vi "Sim_Yoke_Shin_TP059851_SPCC_Assignment_server.vi"() -> ()   [LabVIEW 2020]
uses:
  <vilib>/Utility/file.llb/Read Delimited Spreadsheet (string).vi
  <vilib>/Utility/file.llb/Write Delimited Spreadsheet (string).vi
panel:
  out "Amount out":string
  out "Data from Client":string
  out "error of functions":errorcluster
  out "error of login":errorcluster
  out "user input":string
  out "Output User Details":string
  out "User ID Array":string[](array[string])
  # "Server"
  # "Login"
  # "Functions"
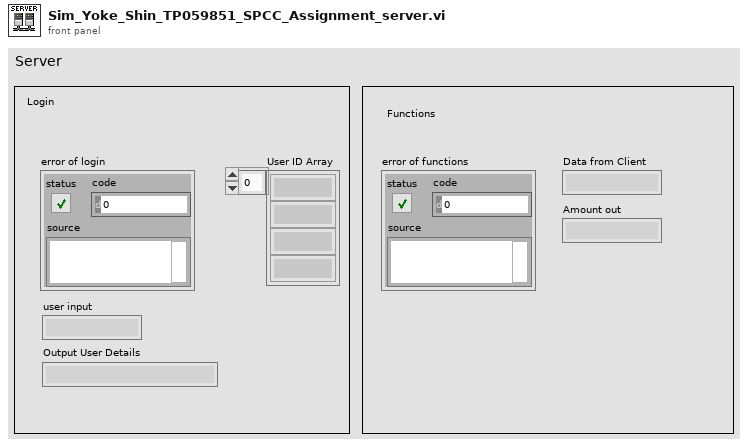
[diagram p1: front panel]
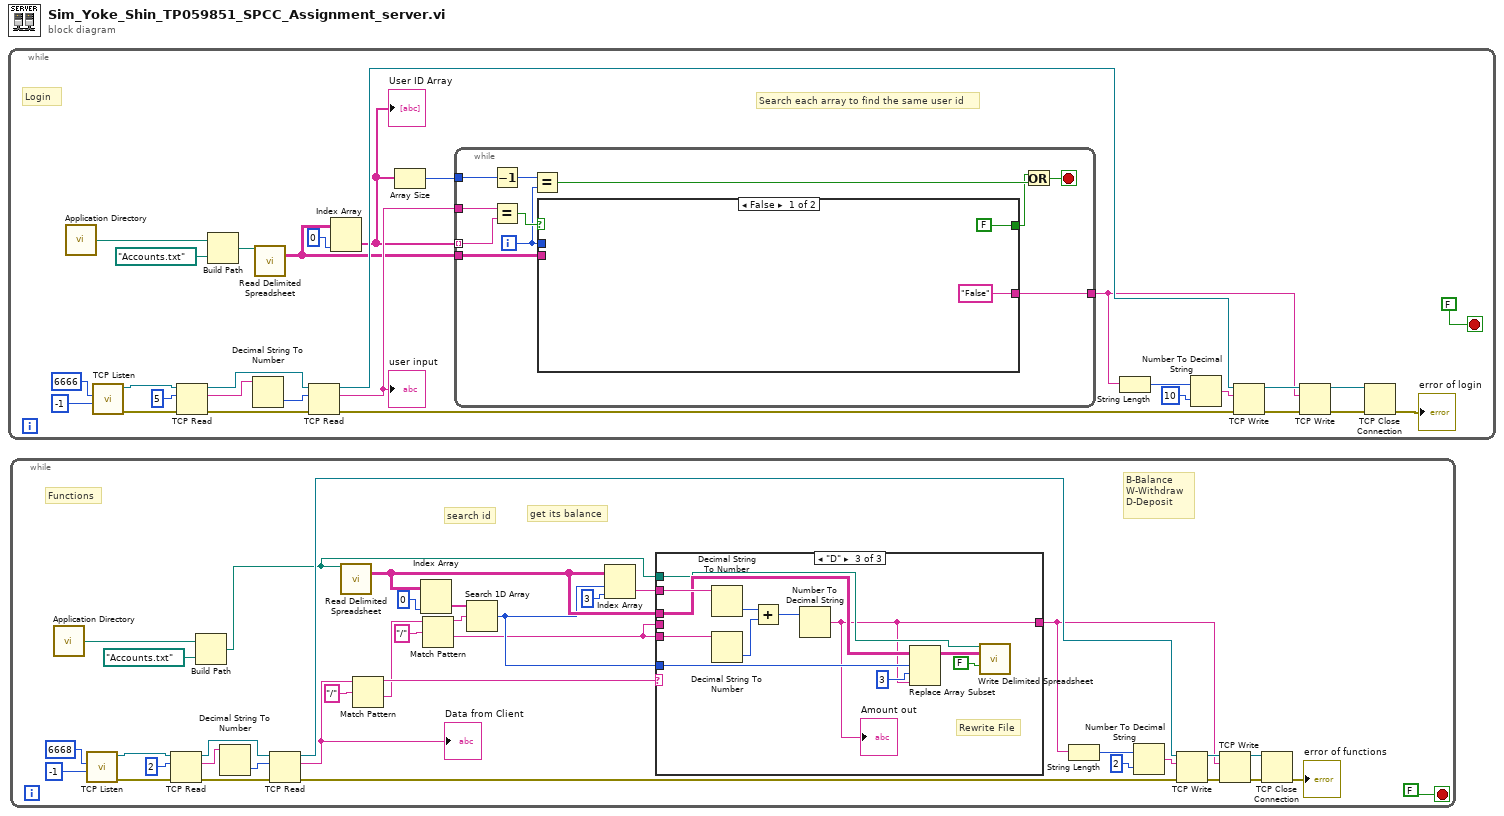
[diagram p0: block diagram]
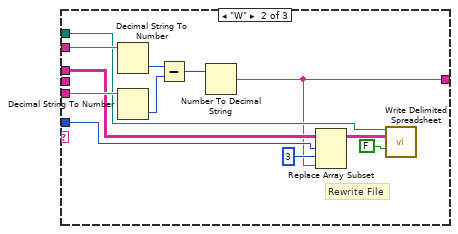
[diagram p3: hidden frame]
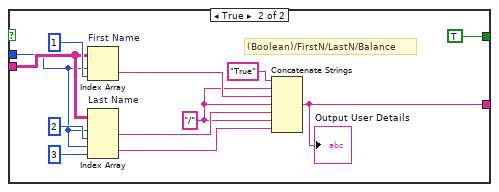
[diagram p4: hidden frame]
diagram:
  n1 = while {
    stop <- FALSE stop-if-true
    # "Search each array to find the same user id"
    # "Login"
    n2 = call <vilib>:"Application Directory.vi"() -> ("Application Directory"=w2:path)
    n3 = call <vilib>:"TCP Listen.vi"("timeout ms (wait forever: -1)"=-1, "port"=u16 6666) -> ("error out"=w20:errorcluster, "connection ID"=w29:refnum<k5>)  [unwired: 5 in, 3 out]
    n4 = TCP Read(connection ID=w29, bytes to read=5, error in (no error)=w20) -> (connection ID out=w28:refnum<k5>, data out=w18:string, error out=w21:errorcluster)  [unwired: 2 in]
    n5 = Build Path(base path=w2, name or relative path=path "Accounts.txt") -> (appended path=w1:path)
    n6 = Decimal String To Number(string=w18) -> (number=w17:i32)  [unwired: 2 in, 1 out]
    n7 = call-poly <vilib>:"Read Delimited Spreadsheet.vi"("file path (dialog if empty)"=w1) -> ("all rows"=w15:string[][])  [unwired: 9 in, 5 out]
    n8 = TCP Read(connection ID=w28, bytes to read=w17, error in (no error)=w21) -> (connection ID out=w27:refnum<k5>, data out=w16:string, error out=w22:errorcluster)  [unwired: 2 in]
    "user input" <- w16
    n9 = Index Array(array=w15, index (col)=0 ("disabled index (col)")) -> (element=w14:string[])  [unwired: 1 in]
    "User ID Array" <- w14
    n10 = Array Size(array=w14) -> (size(s)=w10:i32)
    n11 = while {
      tunnel: w14 -> [w33] mode=indexing
      tunnel: w16 -> [w39]
      tunnel: w15 -> [w38]
      tunnel: [w34] -> w13
      tunnel: w10 -> [w32]
      i -> [w36]
      stop <- w30 stop-if-true
      n12 = Decrement(x=w32) -> (x-1=w37:i32)
      n13 = Equal?(x=w39, y=w33) -> (x = y?=w40:bool)
      n14 = Equal?(x=w37, y=w36) -> (x = y?=w35:bool)
      n15 = case shown="False" w40 {
        tunnel: w38 -> [_ w47]
        tunnel: w36 -> [_ w46]
        tunnel: [FALSE TRUE] -> w31
        tunnel: ["False" w48] -> w34
        frame False {
        }
        frame True {
          w44 = "/" ("string")
          # "(Boolean)/FirstN/LastN/Balance"
          n16 = Index Array "First Name"(array=w47, index (row)=w46, index (col)=1 ("disabled index (col)")) -> (element=w50:string)
          n17 = Index Array "Last Name"(array=w47, index (row) #1=w46, index (col) #1=2 ("disabled index (col)"), index (row) #2=w46, index (col) #2=3 ("disabled index (col)")) -> (element #1=w49:string, element #2=w43:string)
          n18 = Concatenate Strings("True" ("string"), w44, w50, w44, w49, w44, w43) -> (w48:string)
          "Output User Details" <- w48
        }
      }
      n19 = Or(x=w31, y=w35) -> (x .or. y?=w30:bool)
    }
    n20 = String Length(string=w13) -> (length=w12:i32)
    n21 = Number To Decimal String(number=w12, width (-)=i16 10) -> (decimal integer string=w11:string)
    n22 = TCP Write(connection ID=w27, data in=w11, error in (no error)=w22) -> (connection ID out=w26:refnum<k5>, error out=w23:errorcluster)  [unwired: 1 in, 1 out]
    n23 = TCP Write(connection ID=w26, data in=w13, error in (no error)=w23) -> (connection ID out=w25:refnum<k5>, error out=w24:errorcluster)  [unwired: 1 in, 1 out]
    n24 = TCP Close Connection(connection ID=w25, error in (no error)=w24) -> (error out=→"error of login":errorcluster)  [unwired: 1 in, 1 out]
  }
  n25 = while {
    stop <- FALSE stop-if-true
    # "B-Balance\nW-Withdraw\nD-Deposit"
    # "Functions"
    # "get its balance"
    # "search id"
    n26 = call <vilib>:"Application Directory.vi"() -> ("Application Directory"=w58:path)
    n27 = call <vilib>:"TCP Listen.vi"("timeout ms (wait forever: -1)"=-1, "port"=u16 6668) -> ("error out"=w81:errorcluster, "connection ID"=w91:refnum<k5>)  [unwired: 5 in, 3 out]
    n28 = TCP Read(connection ID=w91, bytes to read=2, error in (no error)=w81) -> (connection ID out=w90:refnum<k5>, data out=w77:string, error out=w82:errorcluster)  [unwired: 2 in]
    n29 = Build Path(base path=w58, name or relative path=path "Accounts.txt") -> (appended path=w56:path)
    n30 = Decimal String To Number(string=w77) -> (number=w76:i32)  [unwired: 2 in, 1 out]
    n31 = TCP Read(connection ID=w90, bytes to read=w76, error in (no error)=w82) -> (connection ID out=w89:refnum<k5>, data out=w55:string, error out=w83:errorcluster)  [unwired: 2 in]
    "Data from Client" <- w55
    n32 = call-poly <vilib>:"Read Delimited Spreadsheet.vi"("file path (dialog if empty)"=w56) -> ("all rows"=w66:string[][])  [unwired: 9 in, 5 out]
    n33 = Match Pattern(string=w55, regular expression="/") -> (before substring=w73:string, after substring=w72:string)  [unwired: 1 in, 2 out]
    n34 = Index Array(array=w66, index (col)=0 ("disabled index (col)")) -> (element=w75:string[])  [unwired: 1 in]
    n35 = Match Pattern(string=w72, regular expression="/") -> (before substring=w70:string, after substring=w60:string)  [unwired: 1 in, 2 out]
    n36 = Search 1D Array(1D array=w75, element=w70) -> (index of element=w65:i32)  [unwired: 1 in]
    n37 = Index Array(array=w66, index (row)=w65, index (col)=3 ("disabled index (col)")) -> (element=w67:string)
    n38 = case shown="\"D\"" w73 {
      tunnel: w67 -> [w92 w99 w116]
      tunnel: w60 -> [_ _ _]
      tunnel: w66 -> [_ w97 w112]
      tunnel: w65 -> [_ w94 w111]
      tunnel: w56 -> [_ w95 w108]
      tunnel: [w92 w93 w106] -> w64
      tunnel: w60 -> [_ w98 w105]
      frame "B", Default {
      }
      frame "W" {
        # "Rewrite File"
        n39 = Decimal String To Number(string=w99) -> (number=w104:i32)  [unwired: 2 in, 1 out]
        n40 = Decimal String To Number(string=w98) -> (number=w103:i32)  [unwired: 2 in, 1 out]
        n41 = Subtract(x=w104, y=w103) -> (x-y=w102:i32)
        n42 = Number To Decimal String(number=w102) -> (decimal integer string=w93:string)  [unwired: 1 in]
        n43 = Replace Array Subset(array=w97, new element=w93, index (row)=w94, index (col)=3 ("disabled index (col)")) -> (w96:string[][])
        n44 = call-poly <vilib>:"Write Delimited Spreadsheet.vi"("file path (dialog if empty)"=w95, "2D data"=w96, "append to file? (new file:F)"=FALSE) -> ()  [unwired: 11 in, 2 out]
      }
      frame "D" {
        # "Rewrite File"
        n45 = Decimal String To Number(string=w116) -> (number=w115:i32)  [unwired: 2 in, 1 out]
        n46 = Decimal String To Number(string=w105) -> (number=w114:i32)  [unwired: 2 in, 1 out]
        n47 = Add(x=w115, y=w114) -> (x+y=w113:i32)
        n48 = Number To Decimal String(number=w113) -> (decimal integer string=w106:string)  [unwired: 1 in]
        "Amount out" <- w106
        n49 = Replace Array Subset(array=w112, new element=w106, index (row)=w111, index (col)=3 ("disabled index (col)")) -> (w109:string[][])
        n50 = call-poly <vilib>:"Write Delimited Spreadsheet.vi"("file path (dialog if empty)"=w108, "2D data"=w109, "append to file? (new file:F)"=FALSE) -> ()  [unwired: 11 in, 2 out]
      }
    }
    n51 = String Length(string=w64) -> (length=w63:i32)
    n52 = Number To Decimal String(number=w63, width (-)=i16 2) -> (decimal integer string=w62:string)
    n53 = TCP Write(connection ID=w89, data in=w62, error in (no error)=w83) -> (connection ID out=w88:refnum<k5>, error out=w84:errorcluster)  [unwired: 1 in, 1 out]
    n54 = TCP Write(connection ID=w88, data in=w64, error in (no error)=w84) -> (connection ID out=w87:refnum<k5>, error out=w85:errorcluster)  [unwired: 1 in, 1 out]
    n55 = TCP Close Connection(connection ID=w87, error in (no error)=w85) -> (error out=→"error of functions":errorcluster)  [unwired: 1 in, 1 out]
  }
